vi "Configure Offset and Limits (Spectrum Emission Mask - Frequency).vi"(0 "VISA resource name":refnum<visa-resource-name>, 7 "Manual Start Frequency List":dbl[](array[numeric])=[2515000.0, 2515000.0, 2515000.0, 2515000.0, 2515000.0] format="%#.6g", 9 "Stop Frequency List":dbl[](array[numeric])=[2715000.0, 2715000.0, 2715000.0, 2715000.0, 2715000.0] format="%#.6g", 11 "error in (no error)":errorcluster) -> (4 "VISA resource name out":refnum<visa-resource-name>, 15 "error out":errorcluster)   [LabVIEW 2022 SP3, in "Agilent N934X Series.lvlib"]
doc: "Configures the frequency and offset side settings under the offsets and limits for Spectrum Emission Mask measurement type.\n\nNote:\nThis VI is only applicable for N9321C, N9322C, N9323C, N9324C models."
uses:
  <instrlib>/Agilent N934X Series/Agilent N934X Series.lvlib
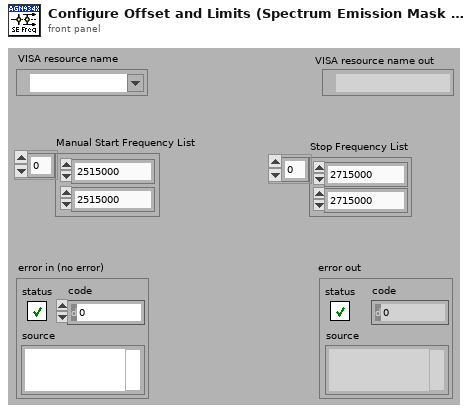
[diagram p1: front panel]
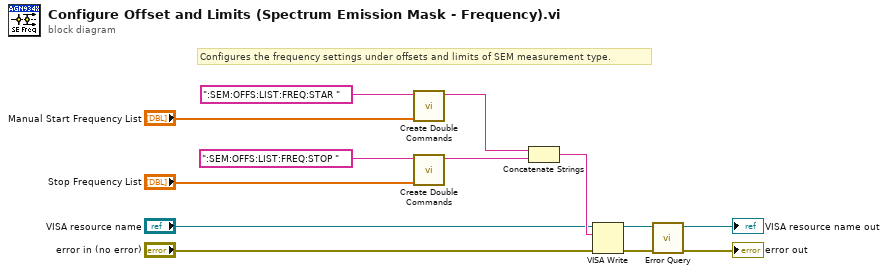
[diagram p0: block diagram]
diagram:
  # "Configures the frequency settings under offsets and limits of SEM measurement type."
  n1 = call <instrlib>:"Create Double Commands.vi"("Double Values"="Manual Start Frequency List", "Commands"=":SEM:OFFS:LIST:FREQ:STAR " ("format string")) -> ("Result"=w3:string)  [unwired: 9 in]
  n2 = call <instrlib>:"Create Double Commands.vi"("Double Values"="Stop Frequency List", "Commands"=":SEM:OFFS:LIST:FREQ:STOP " ("format string")) -> ("Result"=w4:string)  [unwired: 9 in]
  n3 = Concatenate Strings(w3, w4) -> (w13:string)
  n4 = VISA Write(VISA resource name="VISA resource name", write buffer=w13, error in (no error)="error in (no error)") -> (VISA resource name out=w7:refnum<visa-resource-name>, error out=w8:errorcluster)  [unwired: 1 out]
  n5 = call <instrlib>:"Error Query.vi"("error in (no error)"=w8, "VISA resource name"=w7) -> ("error out"=→"error out":errorcluster, "VISA resource name out"=→"VISA resource name out":refnum<visa-resource-name>)  [unwired: 6 in, 2 out]
